vi "Weather Simulator.vi"(11 "error in (no error)":errorcluster) -> (6 "Waveform Graph":dynamicdata(graph), 15 "error out":errorcluster)   [LabVIEW 2010]
doc: "This VI generated a temperature reading and a voltage reading on a sine wave at 50kHz for 5000 points. This VI is used as a simulation in the Weather Station project when no hardware is available."
uses:
  Instance           2 25Saved   Weather Simulator .vi
  Instance           1 25Saved   Weather Simulator .vi
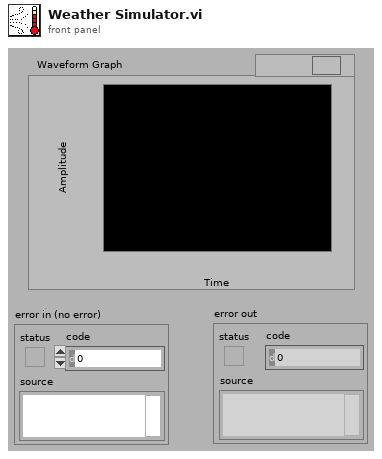
[diagram p1: front panel]
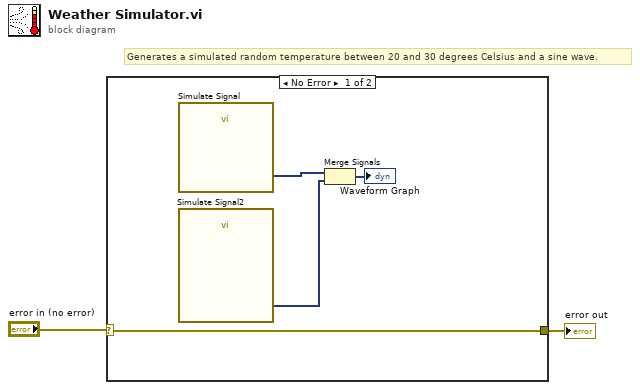
[diagram p0: block diagram]
diagram:
  # "Generates a simulated random temperature between 20 and 30 degrees Celsius and a sine wave."
  n1 = case shown="No Error" "error in (no error)" {
    selector: "error in (no error)" -> [w6 w7]
    tunnel: [w6 w7] -> w1
    frame No Error {
      n2 = call "Simulate Signal"() -> ("Temperature"=w5:dynamicdata)  [unwired: 14 in, 1 out]
      n3 = call "Simulate Signal2"() -> ("Sine"=w4:dynamicdata)  [unwired: 14 in, 1 out]
      n4 = Merge Signals(w5, w4) -> (→"Waveform Graph":dynamicdata)
    }
    frame Error {
    }
  }
  "error out" <- w1
